vi "FGV - Alazar Data Buffer.vi"(7 "Actions":T1, 8 "error in (no error)":errorcluster, 10 "ASync Read Parameters":T2, 11 "Array In":sgl[](array[numeric])) -> (0 "error out":errorcluster, 3 "Array Out":sgl[](array[numeric]))   [LabVIEW 2018]
uses:
  Controls/Async Read Parameters.ctl
  General/Controls/FGV Actions.ctl
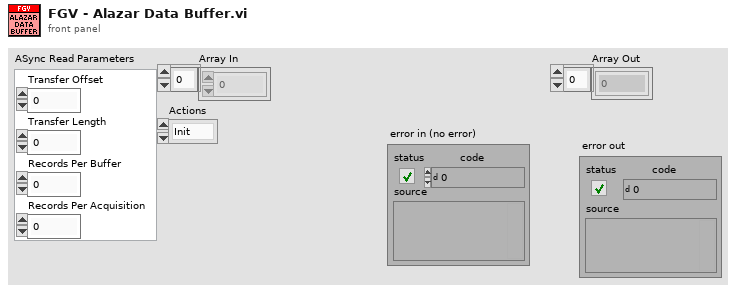
[diagram p1: front panel]
types:
  T1 = typedef "FGV Actions.ctl" = enum16{"Init", "Set", "Get", "Clear"}
  T2 = typedef "Async Read Parameters.ctl" = cluster{"Transfer Offset":u32, "Transfer Length":u32, "Records Per Buffer":u32, "Records Per Acquisition":u32}
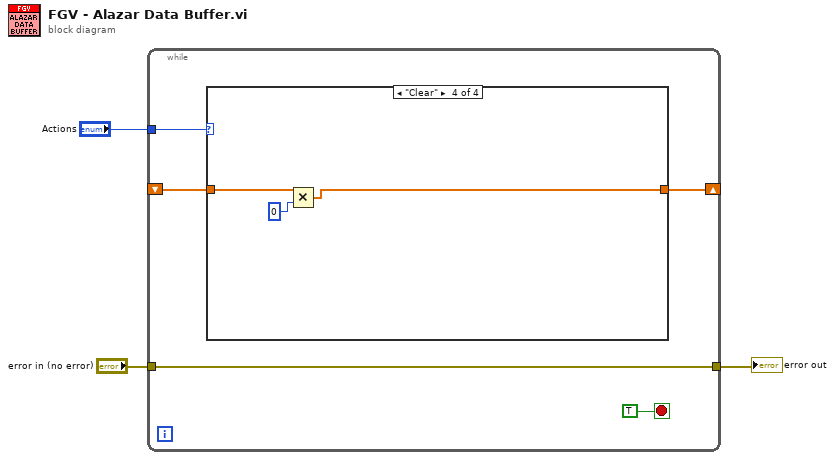
[diagram p0: block diagram]
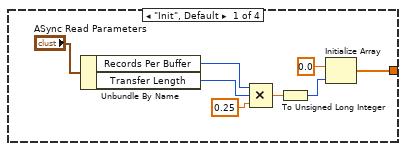
[diagram p2: hidden frame]
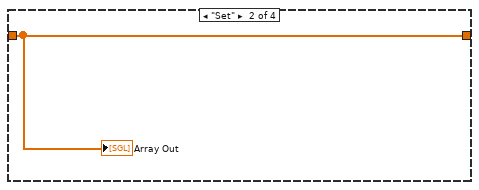
[diagram p3: hidden frame]
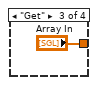
[diagram p4: hidden frame]
diagram:
  n1 = while {
    tunnel: "Actions" -> [w7]
    shift-right: [w6] -> _
    shift-left: _ -> [w5]
    tunnel: [w4] -> w1
    tunnel: "error in (no error)" -> [w4]
    stop <- TRUE stop-if-true
    n2 = case shown="\"Clear\"" w7 {
      tunnel: [w9 w17 "Array In" w19] -> w6
      tunnel: w5 -> [_ w17 _ w21]
      frame "Init", Default {
        n3 = Unbundle By Name("ASync Read Parameters") -> ("Records Per Buffer"=w15:u32, "Transfer Length"=w12:u32)
        n4 = Compound Arithmetic op=MULTIPLY(w15, w12, 0.25 ("y")) -> (w16:dbl)
        n5 = To Unsigned Long Integer(number=w16) -> (unsigned 32bit integer=w10:u32)
        n6 = Initialize Array(sgl 0.0, w10) -> (w9:sgl[])
      }
      frame "Set" {
        "Array Out" <- w17
      }
      frame "Get" {
      }
      frame "Clear" {
        n7 = Multiply(x=w21, y=0) -> (x*y=w19:sgl[])
      }
    }
  }
  "error out" <- w1
